vi "Save Images.vi"(6 "Step Number":i32, 8 "error in (no error)":errorcluster, 9 "Image Name":string, 10 "Image":T1, 11 "Directory":path) -> (0 "error out":errorcluster, 2 "Image Path":path, 3 "Dup Directory out":path)   [LabVIEW 2020, in "MacroAssert.lvlib" / "Image Assertion.lvclass"]
doc: "Saves <B>Expected Image</B> and <B>Actual Image</B> to file."
uses:
  Image Assertion.lvclass
  Image Assertion.lvclass/Image Assertion.ctl
  <vilib>/picture/picture.llb/imagedata.ctl
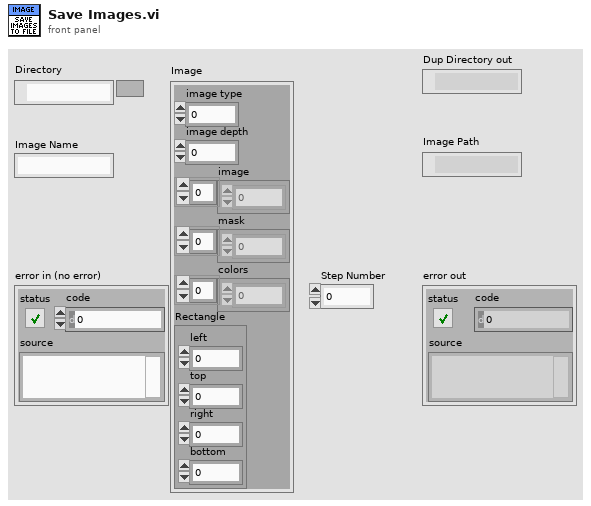
[diagram p1: front panel]
types:
  T1 = typedef "imagedata.ctl" = cluster{"image type":i32, "image depth":i32, "image":u8[], "mask":u8[], "colors":u32[], "Rectangle":cluster{"left":i16, "top":i16, "right":i16, "bottom":i16}}
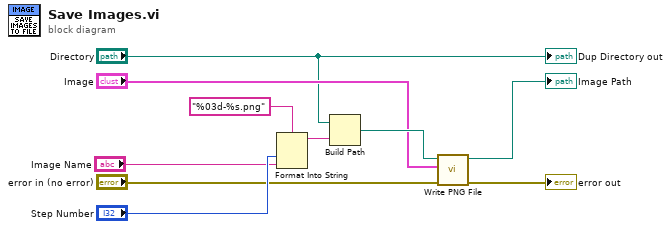
[diagram p0: block diagram]
diagram:
  n1 = Format Into String(format string="%03d-%s.png", "Step Number", "Image Name") -> (resulting string=w8:string)  [unwired: 2 in, 1 out]
  n2 = Build Path(base path="Directory", name or relative path=w8) -> (appended path=w7:path)
  n3 = call <vilib>:"Write PNG File.vi"("error in (no error)"="error in (no error)", "image data"="Image", "path to PNG file"=w7) -> ("error out"=→"error out":errorcluster, "path"=→"Image Path":path)  [unwired: 7 in]
  "Dup Directory out" <- "Directory"
